vi "7SegmentReservoir.vi"() -> ()   [LabVIEW 2020]
panel:
  out "Danger":bool
  out "Normal":bool
  in  "D --":dbl(slide) scale=0.0..99.0
  in  "D ++":dbl(slide) scale=0.0..99.0
  out "Réservoir d'eau":dbl(slide) scale=0.0..99.0
  out "C 2":bool
  out "E 2":bool
  out "D 2":bool
  out "B  2":bool
  out "G 2":bool
  out "F 2":bool
  out "A 2":bool
  out "C":bool
  out "E":bool
  out "D":bool
  out "B":bool
  out "G":bool
  out "F":bool
  out "A":bool
  in  "stop":bool
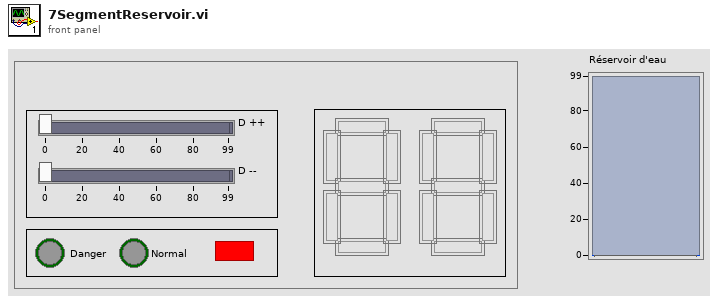
[diagram p1: front panel]
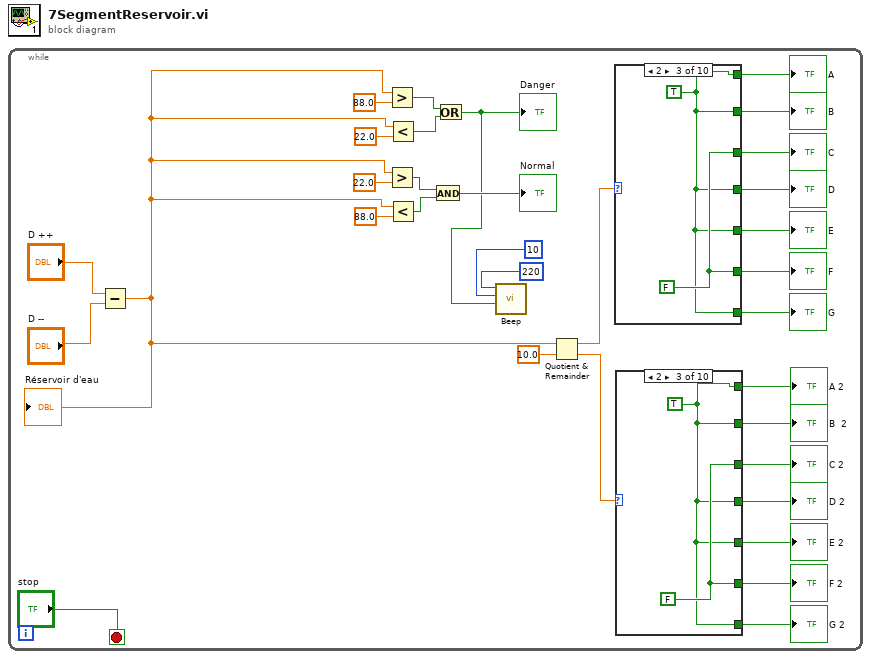
[diagram p0: block diagram]
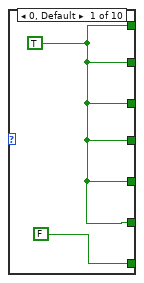
[diagram p2: hidden frame]
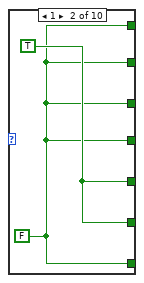
[diagram p3: hidden frame]
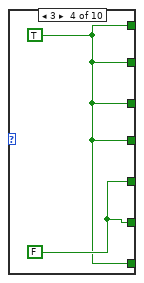
[diagram p4: hidden frame]
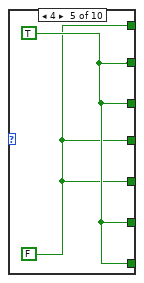
[diagram p5: hidden frame]
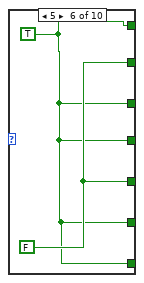
[diagram p6: hidden frame]
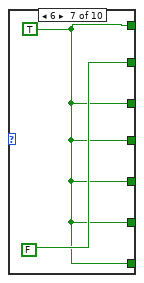
[diagram p7: hidden frame]
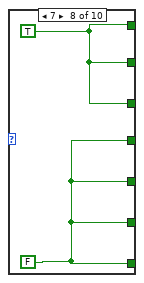
[diagram p8: hidden frame]
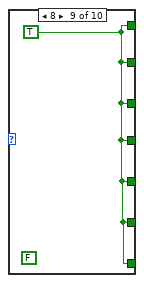
[diagram p9: hidden frame]
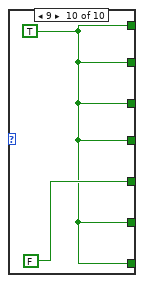
[diagram p10: hidden frame]
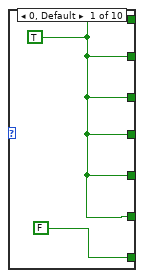
[diagram p11: hidden frame]
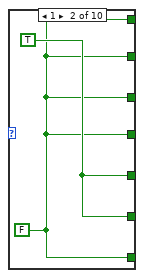
[diagram p12: hidden frame]
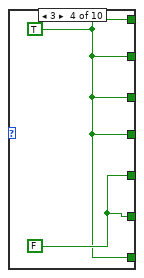
[diagram p13: hidden frame]
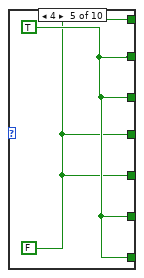
[diagram p14: hidden frame]
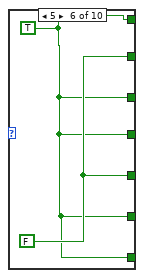
[diagram p15: hidden frame]
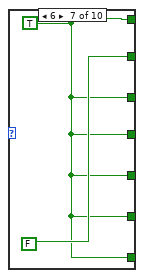
[diagram p16: hidden frame]
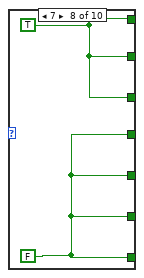
[diagram p17: hidden frame]
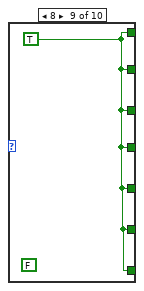
[diagram p18: hidden frame]
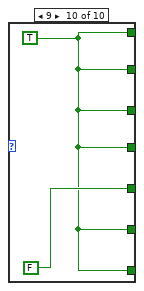
[diagram p19: hidden frame]
diagram:
  n1 = while {
    stop <- "stop" stop-if-true
    n2 = Subtract(x="D ++", y="D --") -> (x-y=w4:dbl)
    "Réservoir d'eau" <- w4
    n3 = Greater?(x=w4, y=88.0) -> (0:w10:bool)
    n4 = Greater?(x=w4, y=22.0) -> (0:w11:bool)
    n5 = Less?(x=w4, y=22.0) -> (x < y?=w13:bool)
    n6 = Less?(x=w4, y=88.0) -> (x < y?=w12:bool)
    n7 = And(x=w11, y=w12) -> (x .and. y?=→"Normal":bool)
    n8 = Or(x=w10, y=w13) -> (x .or. y?=w1:bool)
    "Danger" <- w1
    n9 = call <vilib>:"Beep.vi"("use system alert? (T)"=w1, "duration (msec)"=u32 10, "frequency (Hz)"=u32 220) -> ()  [unwired: 9 in]
    n10 = Quotient & Remainder(x=w4, y=10.0) -> (x-y*floor(x/y)=w17:dbl, floor(x/y)=w16:dbl)
    n11 = case shown="2" w17 {
      tunnel: [w53 w55 w57 w59 w61 w63 w65 w68 w69 w70] -> w32
      tunnel: [w53 w55 w57 w59 w62 w64 FALSE w68 w69 w70] -> w31
      tunnel: [w53 w55 w58 w59 w62 w63 w65 w68 w69 w70] -> w30
      tunnel: [w53 w55 w57 w59 w61 w63 w65 w67 w69 w70] -> w29
      tunnel: [w53 w56 w57 w60 w61 w64 w65 w67 w69 FALSE] -> w28
      tunnel: [w53 w56 w58 w60 w62 w63 w65 w67 w69 w70] -> w27
      tunnel: [FALSE w55 w57 w59 w62 w63 w65 w67 w69 w70] -> w26
      frame 0, Default {
        w53 = TRUE
      }
      frame 1 {
        w55 = FALSE
        w56 = TRUE
      }
      frame 2 {
        w58 = FALSE
        w57 = TRUE
      }
      frame 3 {
        w60 = FALSE
        w59 = TRUE
      }
      frame 4 {
        w61 = FALSE
        w62 = TRUE
      }
      frame 5 {
        w64 = FALSE
        w63 = TRUE
      }
      frame 6 {
        w65 = TRUE
      }
      frame 7 {
        w67 = FALSE
        w68 = TRUE
      }
      frame 8 {
        (unwired) FALSE
        w69 = TRUE
      }
      frame 9 {
        w70 = TRUE
      }
    }
    "A" <- w32
    "F" <- w27
    "G" <- w26
    "B" <- w31
    "D" <- w29
    "E" <- w28
    "C" <- w30
    n12 = case shown="2" w16 {
      tunnel: [w34 w36 w38 w40 w42 w44 w46 w49 w50 w51] -> w24
      tunnel: [w34 w36 w38 w40 w43 w45 FALSE w49 w50 w51] -> w23
      tunnel: [w34 w36 w39 w40 w43 w44 w46 w49 w50 w51] -> w22
      tunnel: [w34 w36 w38 w40 w42 w44 w46 w48 w50 w51] -> w21
      tunnel: [w34 w37 w38 w41 w42 w45 w46 w48 w50 FALSE] -> w20
      tunnel: [w34 w37 w39 w41 w43 w44 w46 w48 w50 w51] -> w19
      tunnel: [FALSE w36 w38 w40 w43 w44 w46 w48 w50 w51] -> w18
      frame 0, Default {
        w34 = TRUE
      }
      frame 1 {
        w36 = FALSE
        w37 = TRUE
      }
      frame 2 {
        w39 = FALSE
        w38 = TRUE
      }
      frame 3 {
        w41 = FALSE
        w40 = TRUE
      }
      frame 4 {
        w42 = FALSE
        w43 = TRUE
      }
      frame 5 {
        w45 = FALSE
        w44 = TRUE
      }
      frame 6 {
        w46 = TRUE
      }
      frame 7 {
        w48 = FALSE
        w49 = TRUE
      }
      frame 8 {
        (unwired) FALSE
        w50 = TRUE
      }
      frame 9 {
        w51 = TRUE
      }
    }
    "A 2" <- w24
    "F 2" <- w19
    "G 2" <- w18
    "B  2" <- w23
    "D 2" <- w21
    "E 2" <- w20
    "C 2" <- w22
  }
